vi "ziExample-HF2-Noise.vi"() -> ()   [LabVIEW 2009]
doc: "Control a Zurich instrument device via the LabOne Labview API. \nRequirements: Zurich Instruments HF2.\n\nThis is an example for a Zurich Instruments HF2 instrument. This example VI calculates the rms noise and the noise spectral densitiy of the input signal at a certain demodulator frequency. \n\nThe VI performs the following steps:\n(1) Load the settings file or, adjust the required settings in ziControl. Set the required demodulator frequency and the required time constant / bandwidth. \n(2) the VI subrscribes to the corresponding demodulator (this demodulator needs to be switched on in the user manual, otherwise no data is received) \n(3) the data is acquired/polled and the RMS noise is calculated by using the following equation:\n RMSnoise = RMS(X - Xmean), RMS stands for root-mean-square\n the number of averages can be chosen by the user \n\n© Zurich Instruments AG, www.zhinst.com"
uses:
  <instrlib>/Zurich Instruments LabOne/Public/Configure/ziGetValueDouble.vi
  <vilib>/measure/madcrms.llb/Basic Averaged DC-RMS for 1 Chan.vi
  <instrlib>/Zurich Instruments LabOne/Public/Data/ziGetEventDemodSample.vi
  <instrlib>/Zurich Instruments LabOne/Zurich Instruments LabOne.lvlib
  <vilib>/measure/NI_MAPro.lvlib
panel:
  out "Error Out":errorcluster
  out "Sel. Device":string
  in  "Address":string="DEV"
  in  "Averaging":i32=100 min=0 max=1024 step=1
  in  "ReadSettingsFile":bool=TRUE caption="Read Settings File"
  out "BW":dbl=9.729925316888316 format="%#_6p"
  out "Ref Freq [Hz]":dbl=1141592.6499998362 format="%#_6p"
  out "Noise Spectral Density\nVrms/sqrt(Hz)":dbl=1.331104953906021e-08 format="%0.2p"
  in  "X or Y":u16(ring) items=["Xnoise", "Ynoise", "Rnoise"]
  out "RMS Value":dbl(graph)=4.1520928155609186e-08
  out "RMS noise":dbl=4.1520928155609186e-08 format="%0.2p"
  in  "Demodulator":u16(ring) items=["Demod 1", "Demod 2", "Demod 3", "Demod 4", "Demod 5", "Demod 6"]
  in  "stop":bool
  # "HF2 Example Noise Measurement.vi\nRequirements: HF2, ziControl for settings, \nZurich Instruments LabVIEW API. \nsee block diagram for VI description"
  # "Tested Devices:\n- HF2LI\nIncompatible Device:\n- UHFLI (wrong BW calcualtions)"
  # "Settings"
  # "Output"
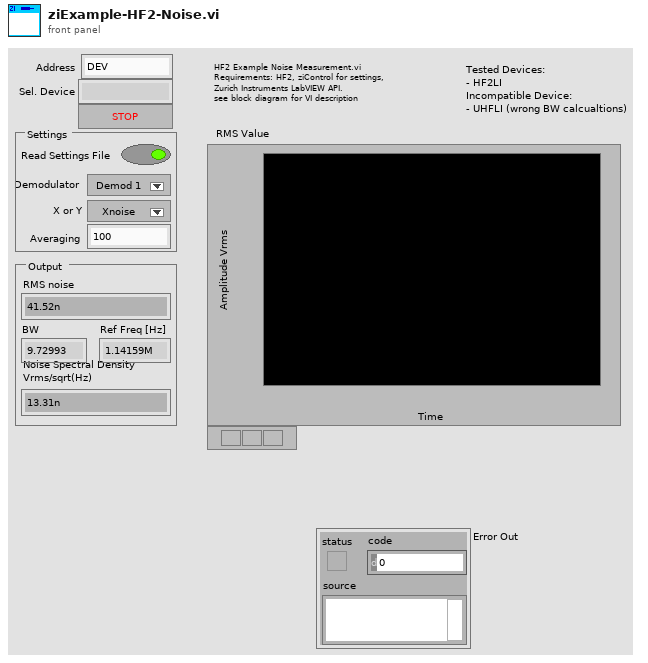
[diagram p1: front panel]
types:
  T1 = typedef "Zurich Instruments LabOne.lvlib/ziTypeHandle.ctl" = cluster{"handleValid":bool, "Conn":u64, "Path Prefix":string, "Handle":u64, "Connected":bool, "Clockbase(s)":dbl}
  T2 = typedef "Zurich Instruments LabOne.lvlib/ziTypeDemodSampleEx.ctl" = cluster{"Timestamps (ticks)":u64[], "X (Vrms)":dbl[], "Y (Vrms)":dbl[], "Osc Phase (rad)":dbl[], "Freq (Hz)":dbl[], "DIO":u32[], "Aux In 0 (V)":dbl[], "Aux In 1 (V)":dbl[], "Trigger":u32[]}
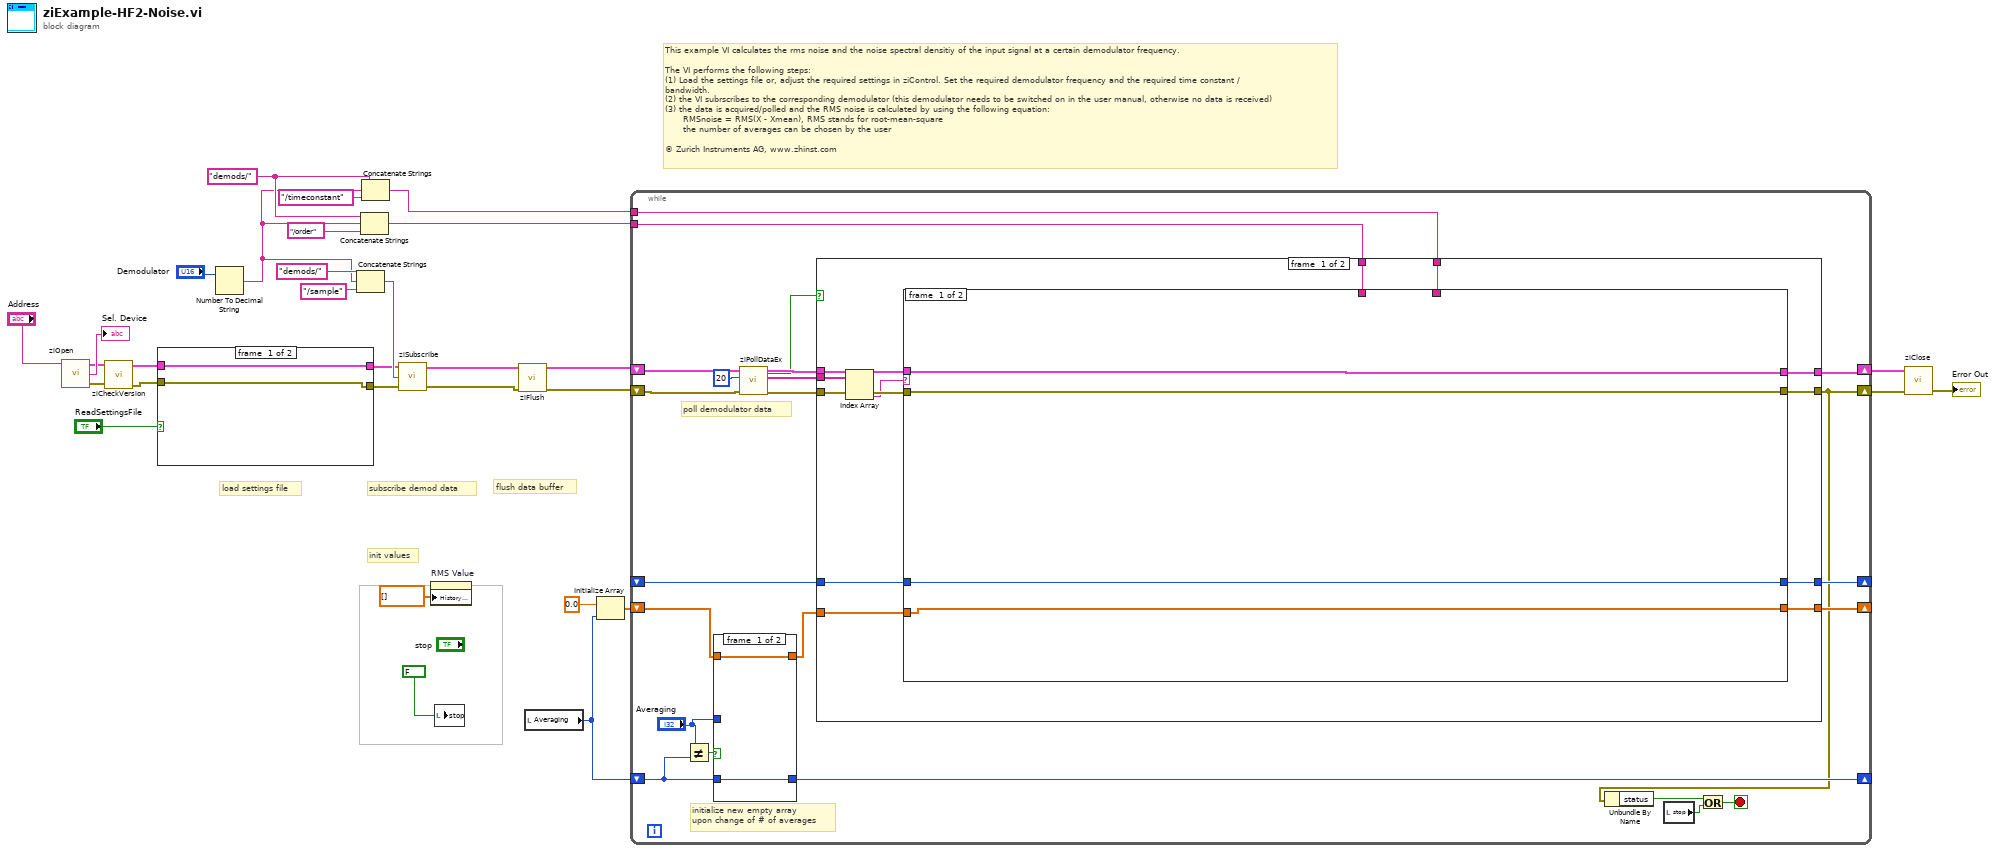
[diagram p0: block diagram]
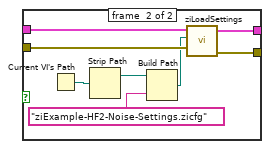
[diagram p2: hidden frame]
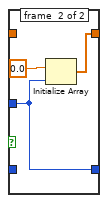
[diagram p3: hidden frame]
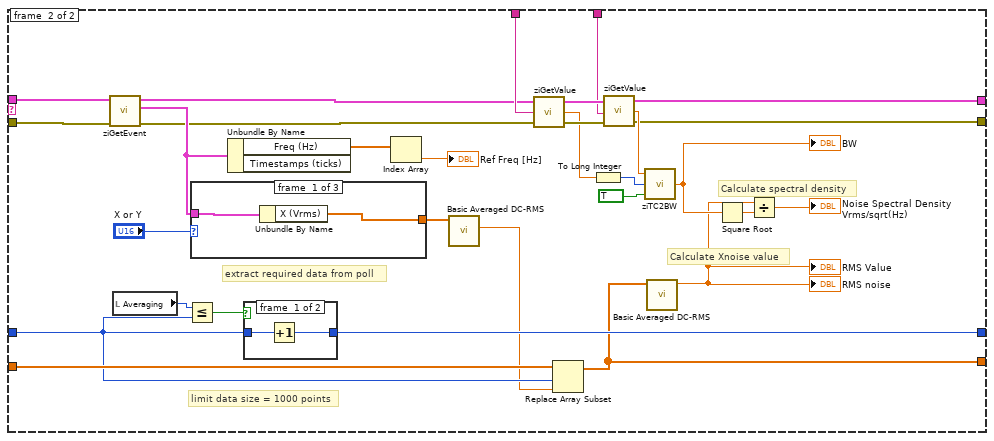
[diagram p4: hidden frame]
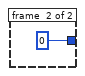
[diagram p5: hidden frame]
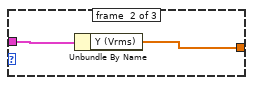
[diagram p6: hidden frame]
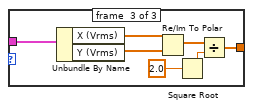
[diagram p7: hidden frame]
diagram:
  w20 = "demods/" ("path")
  # "load settings file"
  # "flush data buffer"
  # "init values"
  # "subscribe demod data"
  # "This example VI calculates the rms noise and the noise spectral densitiy of the input signal at a certain demodulator frequency. \n\nThe VI performs the following steps:\n(1) Load the settings file or, adjust the required settings in ziControl. Set the required demodulator frequency and the required time constant / bandwidth. \n(2) the VI subrscribes to the corresponding demodulator (this demodulator needs to be switched on in the user manual, otherwise no data is received)  \n(3) the data is acquired/polled and the RMS noise is calculated by using the following equation:\n      RMSnoise = RMS(X - Xmean), RMS stands for root-mean-square\n      the number of averages can be chosen by the user \n\n© Zurich Instruments AG, www.zhinst.com"
  n1 = call <instrlib>:"ziOpen.vi"("Address"="Address") -> ("Error Out"=w3:errorcluster, "Selected Device"=→"Sel. Device":string, "HandleOut"=w4:T1)  [unwired: 1 in, 2 out]
  n2 = call <instrlib>:"ziCheckVersion.vi"("Handle In"=w4, "Error In"=w3) -> ("Handle Out"=w1:T1, "Error Out"=w2:errorcluster)  [unwired: 11 in, 1 out]
  n3 = case shown="True" "ReadSettingsFile" {
    tunnel: w1 -> [w33 w41]
    tunnel: w2 -> [w32 w40]
    tunnel: [w33 w39] -> w18
    tunnel: [w32 w38] -> w17
    frame #0 {
    }
    frame #1 {
      n4 = Current VI's Path() -> (path=w34:path)
      n5 = Strip Path(path=w34) -> (stripped path=w35:path)  [unwired: 1 out]
      n6 = Build Path(base path=w35, name or relative path="ziExample-HF2-Noise-Settings.zicfg" ("path")) -> (appended path=w36:path)
      n7 = call <instrlib>:"ziLoadSettings.vi"("Error in"=w40, "File path (dialog if empty)"=w36, "Handle in"=w41) -> ("Error out"=w38:errorcluster, "Handle out"=w39:T1)  [unwired: 2 in]
    }
  }
  n8 = Number To Decimal String(number="Demodulator") -> (decimal integer string=w15:string)  [unwired: 1 out]
  n9 = Concatenate Strings("demods/" ("path"), w15, "/sample" ("path")) -> (w27:string)
  n10 = Concatenate Strings(w20, w15, "/order" ("path")) -> (w25:string)
  n11 = Concatenate Strings(w20, w15, "/timeconstant" ("path")) -> (w24:string)
  n12 = call <instrlib>:"ziSubscribe.vi"("error in"=w17, "Path ()"=w27, "Handle In"=w18) -> ("error out"=w5:errorcluster, "Handle Out"=w8:T1)  [unwired: 1 in]
  n13 = property on="RMS Value" class="WFChart (strict)"("History Data"=dbl[] []) -> ()  [unwired: 2 in, 2 out]
  n14 = local write "stop"(FALSE ("Record")) -> ()
  n15 = call <instrlib>:"ziFlush.vi"("error in"=w5, "Handle In"=w8) -> ("error out"=w6:errorcluster, "Handle Out"=w7:T1)  [unwired: 8 in]
  n16 = local read "Averaging"() -> (w12:i32)
  n17 = Initialize Array(0.0 ("element"), w12) -> (w14:dbl[])
  n18 = while {
    shift-right: [w59] -> w31
    shift-left: w7 -> [w64]
    shift-right: [w44] -> w30
    shift-left: w6 -> [w63]
    shift-right: [w53] -> _
    shift-left: w14 -> [w52]
    tunnel: w25 -> [w57]
    tunnel: w24 -> [w58]
    shift-right: [w54] -> _
    shift-left: _ -> [w55]
    shift-right: [w48] -> _
    shift-left: w12 -> [w47]
    stop <- w42 stop-if-true
    # "initialize new empty array\nupon change of # of averages"
    # "poll demodulator data"
    n19 = Not Equal?(x="Averaging", y=w47) -> (x != y?=w50:bool)
    n20 = case shown="True" w50 {
      tunnel: w52 -> [w66 _]
      tunnel: [w66 w68] -> w51
      tunnel: "Averaging" -> [_ w67]
      tunnel: [w65 w67] -> w48
      tunnel: w47 -> [w65 _]
      frame #0 {
      }
      frame #1 {
        n21 = Initialize Array(0.0 ("element"), w67) -> (w68:dbl[])
      }
    }
    n22 = call <instrlib>:"ziPollDataEx.vi"("error in"=w63, "Timeout ms (50)"=20 ("TimeOut ms (50)"), "Handle In"=w64) -> ("error out"=w60:errorcluster, "PathArray"=w46:string[], "Handle Out"=w61:T1, "Timed Out"=w56:bool)  [unwired: 1 in, 4 out]
    n23 = case shown="False" w56 {
      tunnel: w61 -> [w73 w133]
      tunnel: w60 -> [w72 w132]
      tunnel: [w79 w133] -> w59
      tunnel: [w78 w132] -> w44
      tunnel: w58 -> [w81 _]
      tunnel: w57 -> [w80 _]
      tunnel: [w76 w130] -> w53
      tunnel: w55 -> [w74 w131]
      tunnel: [w77 w131] -> w54
      tunnel: w51 -> [w75 w130]
      tunnel: w46 -> [w71 _]
      frame #0 {
        n24 = Index Array(array=w71) -> (element #2=w70:string)  [unwired: 2 in, 1 out]
        n25 = case shown="\"demods\"" w70 {
          tunnel: w81 -> [_ w110]
          tunnel: w80 -> [_ w105]
          tunnel: [w85 w103] -> w79
          tunnel: [w84 w102] -> w78
          tunnel: [w82 w101] -> w77
          tunnel: [w83 w97] -> w76
          tunnel: w75 -> [w83 w96]
          tunnel: w74 -> [w82 w95]
          tunnel: w73 -> [w85 w90]
          tunnel: w72 -> [w84 w89]
          frame #0 {
          }
          frame #1 {
            # "extract required data from poll"
            # "Calculate spectral density"
            # "Calculate Xnoise value"
            # "limit data size = 1000 points"
            n26 = call-poly <instrlib>:"ziGetEvent.vi"("Error In"=w89, "Handle In"=w90) -> ("Error Out"=w87:errorcluster, "Demod Sample Out"=w88:T2, "Handle Out"=w86:T1)  [unwired: 7 in]
            n27 = local read "Averaging"() -> (w98:i32)
            n28 = Less Or Equal?(x=w98, y=w95) -> (x <= y?=w100:bool)
            n29 = case shown="2" "X or Y" {
              tunnel: w88 -> [w120 w121 w129]
              tunnel: [w119 w122 w125] -> w99
              frame #0 {
                n30 = Unbundle By Name(w120) -> ("X (Vrms)"=w119:dbl[])
              }
              frame #1 {
                n31 = Unbundle By Name(w121) -> ("Y (Vrms)"=w122:dbl[])
              }
              frame #2 {
                n32 = Unbundle By Name(w129) -> ("X (Vrms)"=w128:dbl[], "Y (Vrms)"=w127:dbl[])
                n33 = Re/Im To Polar(2:w127, 3:w128) -> (1:w126:dbl[])  [unwired: 1 out]
                n34 = Square Root(x=2.0) -> (sqrt(x)=w124:dbl)
                n35 = Divide(x=w126, y=w124) -> (x/y=w125:dbl[])
              }
            }
            n36 = Unbundle By Name(w88) -> ("Freq (Hz)"=w104:dbl[])  [unwired: 1 out]
            n37 = case shown="True" w100 {
              tunnel: [w117 u32 0] -> w101
              tunnel: w95 -> [w116 _]
              frame #0 {
                n38 = Increment(x=w116) -> (x+1=w117:u32)
              }
              frame #1 {
              }
            }
            n39 = Index Array(array=w104) -> (element=→"Ref Freq [Hz]":dbl)  [unwired: 1 in]
            n40 = call-poly <vilib>:"Basic Averaged DC-RMS.vi"("signal in"=w99) -> ("RMS value"=w94:dbl)  [unwired: 4 in, 6 out]
            n41 = call-poly <instrlib>:"ziGetValue.vi"("error in"=w87, "Path"=w105, "Handle in"=w86) -> ("error out"=w112:errorcluster, "Value"=w107:dbl, "Handle out"=w111:T1)
            n42 = Replace Array Subset(array=w96, new element=w94, index=w95) -> (w97:dbl[])
            n43 = To Long Integer(number=w107) -> (32bit integer=w109:i32)
            n44 = call-poly <instrlib>:"ziGetValue.vi"("error in"=w112, "Path"=w110, "Handle in"=w111) -> ("error out"=w102:errorcluster, "Value"=w108:dbl, "Handle out"=w103:T1)
            n45 = call <instrlib>:"ziTC2BW.vi"("Eq BW (F)"=TRUE ("Eq BW"), "Order (1)"=w109, "TC (s)"=w108) -> ("BW (Hz)"=w106:dbl)
            "BW" <- w106
            n46 = call-poly <vilib>:"Basic Averaged DC-RMS.vi"("signal in"=w97) -> ("DC value"=w91:dbl)  [unwired: 4 in, 6 out]
            "RMS noise" <- w91
            "RMS Value" <- w91
            n47 = Square Root(x=w106) -> (sqrt(x)=w113:dbl)
            n48 = Divide(x=w91, y=w113) -> (x/y=→"Noise Spectral Density\nVrms/sqrt(Hz)":dbl)
          }
        }
      }
      frame #1 {
      }
    }
    n49 = Unbundle By Name(w44) -> ("status"=w45:bool)
    n50 = local read "stop"() -> (w43:bool)
    n51 = Or(x=w45, y=w43) -> (x .or. y?=w42:bool)
  }
  n52 = call <instrlib>:"ziClose.vi"("Error In"=w30, "Handle In"=w31) -> ("Error Out"=→"Error Out":errorcluster)  [unwired: 3 out]
